vi "tsapp_delete_cyclic_msg_can_win32.vi"(8 "错误输入（无错误）":errorcluster, 10 "数据帧信息":T1 {"ADLC" max=64; "AID" max=536870911}, 11 "AAppChannel":i32(ring) items=["CHN1", "CHN2", "CHN3", "CHN4", "CHN5", "CHN6", "CHN7", "CHN8", "CHN9", "CHN10", "CHN11", "CHN12", "CHN13", "CHN14", "CHN15", "CHN16", "CHN17", "CHN18", "CHN19", "CHN20", "CHN21", "CHN22", "CHN23", "CHN24", "CHN25", "CHN26", "CHN27", "CHN28", "CHN29", "CHN30", "CHN31", "CHN32"]) -> (0 "错误输出":errorcluster, 3 "tsapp_delete_cyclic_msg_can":i32)   [LabVIEW 2016]
uses:
  CAN_FrameInfo.ctl
  TCANProperty.ctl
  SendMsgInfo.ctl
  D:/Program Files (x86)/TOSUN/TSMaster/bin/Data/SDK/lib/x86/TSMaster.dll
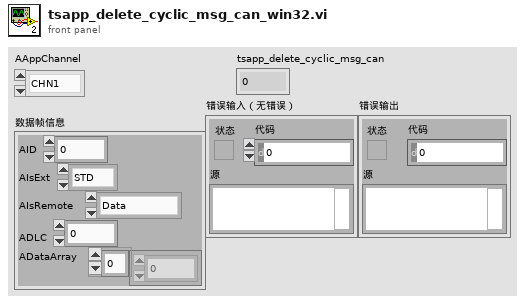
[diagram p1: front panel]
types:
  T1 = typedef "CAN_FrameInfo.ctl" = cluster{"AID":u32, "AIsExt":enum16{"STD", "EXT"}, "AIsRemote":enum16{"Data", "Remote"}, "ADLC":u8, "ADataArray":u8[]}
  T2 = typedef "SendMsgInfo.ctl" = cluster{"FIdxChn":u8, "FProperties":u8, "FDLC":u8, "FReserved":u8, "FIdentifier":i32, "FTimeUS":u64, "Data0":u8, "Data1":u8, "Data2":u8, "Data3":u8, "Data4":u8, "Data5":u8, "Data6":u8, "Data7":u8}
  T3 = typedef "TCANProperty.ctl" = cluster{"istx":bool, "remoteframe":bool, "extframe":bool, "tbd1":bool, "tbd2":bool, "tbd3":bool, "tbd4":bool, "iserrorframe":bool}
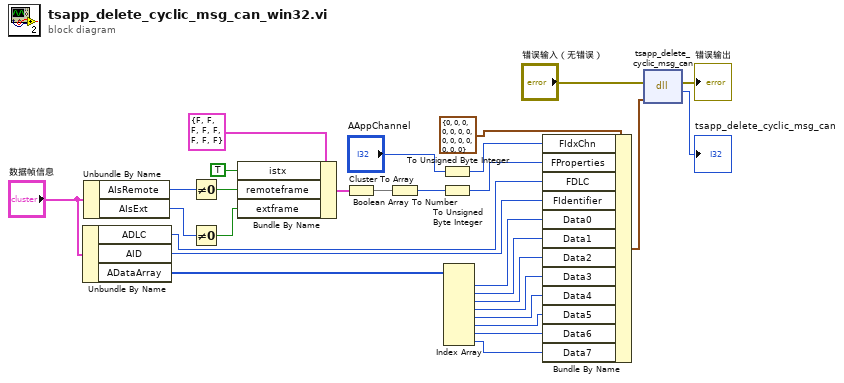
[diagram p0: block diagram]
diagram:
  n1 = Unbundle By Name("数据帧信息") -> ("ADLC"=w17:u8, "AID"=w18:u32, "ADataArray"=w19:u8[])
  n2 = Unbundle By Name("数据帧信息") -> ("AIsRemote"=w10:enum16{"Data", "Remote"}, "AIsExt"=w12:enum16{"STD", "EXT"})
  n3 = Not Equal To 0?(x=w10) -> (x != 0?=w9:bool)
  n4 = Not Equal To 0?(x=w12) -> (x != 0?=w11:bool)
  n5 = Bundle By Name(cluster=T3 {"istx"=FALSE, "remoteframe"=FALSE, "extframe"=FALSE, "tbd1"=FALSE, "tbd2"=FALSE, "tbd3"=FALSE, "tbd4"=FALSE, "iserrorframe"=FALSE} ("TCANProperty"), "istx"=TRUE, "remoteframe"=w9, "extframe"=w11) -> (w13:T3)
  n6 = Cluster To Array(cluster=w13) -> (array=w14:bool[])
  n7 = Boolean Array To Number(Boolean array=w14) -> (number=w15:u32)
  n8 = To Unsigned Byte Integer(number="AAppChannel") -> (unsigned 8bit integer=w6:u8)
  n9 = To Unsigned Byte Integer(number=w15) -> (unsigned 8bit integer=w16:u8)
  n10 = Index Array(array=w19) -> (element #1=w20:u8, element #2=w21:u8, element #3=w22:u8, element #4=w23:u8, element #5=w24:u8, element #6=w25:u8, element #7=w26:u8, element #8=w27:u8)  [unwired: 8 in]
  n11 = Bundle By Name(cluster=T2 {"FIdxChn"=0, "FProperties"=0, "FDLC"=0, "FReserved"=0, "FIdentifier"=0, "FTimeUS"=0, "Data0"=0, "Data1"=0, "Data2"=0, "Data3"=0, "Data4"=0, "Data5"=0, "Data6"=0, "Data7"=0} ("SendMsgInfo"), "FIdxChn"=w6, "FProperties"=w16, "FDLC"=w17, "FIdentifier"=w18, "Data0"=w20, "Data1"=w21, "Data2"=w22, "Data3"=w23, "Data4"=w24, "Data5"=w25, "Data6"=w26, "Data7"=w27) -> (w28:T2)
  n12 = dll-call lib="D:/Program Files (x86)/TOSUN/TSMaster/bin/Data/SDK/lib/x86/TSMaster.dll" fn="tsapp_delete_cyclic_msg_can"(error in="错误输入（无错误）", "ACAN"=w28) -> (error out=→"错误输出":errorcluster, "tsapp_delete_cyclic_msg_can"=→"tsapp_delete_cyclic_msg_can":i32)  [unwired: 3 in, 1 out]
